vi "TestStand, Set Step Limits.vi"(6 "TS index":i32, 8 "error in":errorcluster, 10 "CDT_type":T1={"Measurement Name"="Signal_1", "Result"=3.0, "Low Limit"=-5.0, "High Limit"=5.0, "Units"="mV", "Comp"="GELE", "DataFmt"="%.3f", "LimitFmt"="%.4f"} {"Result" format="%.3g"; "High Limit" format="%.3g"; "Low Limit" format="%.3g"}, 11 "Sequence Context":refnum<k7>) -> (0 "error out":errorcluster, 3 "Sequence Context Out":refnum<k7>)   [LabVIEW 2010]
doc: "Sets TestStand Multiple Numeric Test properties for the following:\n\nRunState.Step.Result.Measurement[index]\nRunState.Step.Result.Measurement[index].Limits.High\nRunState.Step.Result.Measurement[index].Limits.Low\nRunState.Step.Result.Measurement[index].Limits.Units\nRunState.Step.Result.Measurement[index].Limits.Comp"
uses:
  TestStand_Result Control.ctl
  <vilib>/addons/TestStand/_TSUtility.llb/TestStand - Get Property Value (Object).vi
  <vilib>/addons/TestStand/_TSUtility.llb/TestStand - Set Property Value (String).vi
  <vilib>/addons/TestStand/_TSUtility.llb/TestStand - Set Property Value (Number).vi
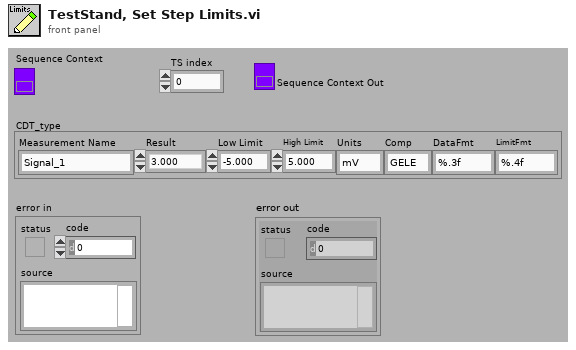
[diagram p1: front panel]
types:
  T1 = typedef "TestStand_Result Control.ctl" = cluster{"Measurement Name":string, "Result":dbl, "Low Limit":dbl, "High Limit":dbl, "Units":string, "Comp":string, "DataFmt":string, "LimitFmt":string}
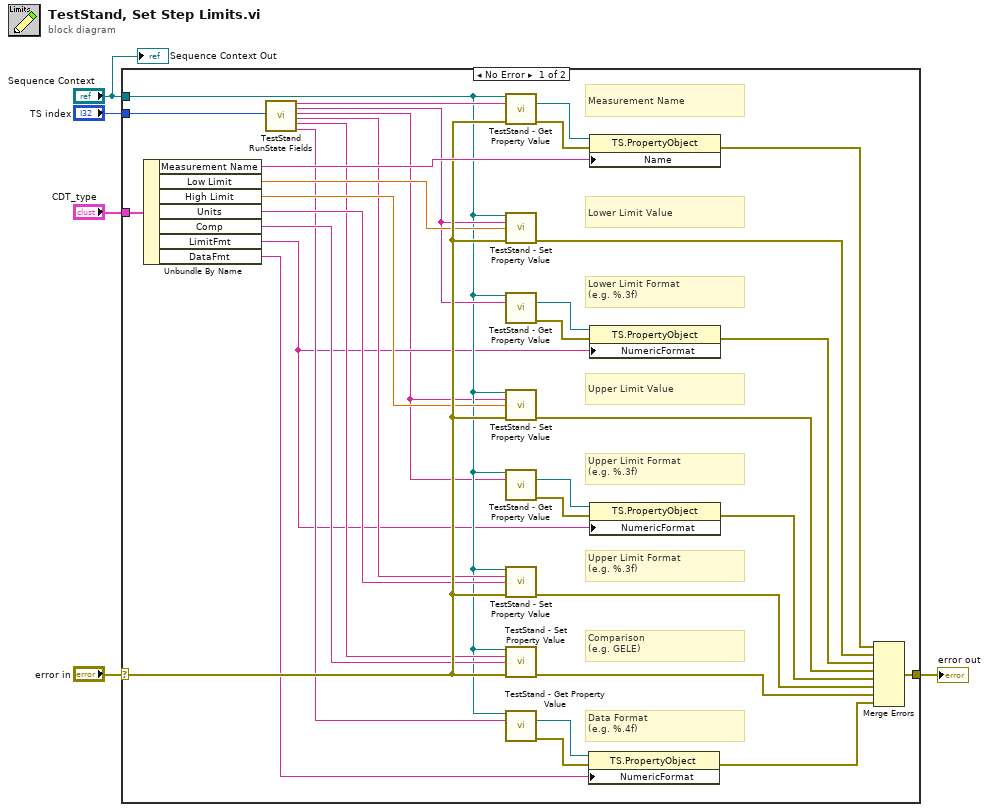
[diagram p0: block diagram]
diagram:
  n1 = case shown="No Error" "error in" {
    selector: "error in" -> [w32 w40]
    tunnel: [w34 w40] -> w5
    tunnel: "Sequence Context" -> [w12 _]
    tunnel: "CDT_type" -> [w33 _]
    tunnel: "TS index" -> [w23 _]
    frame No Error {
      # "Data Format\n(e.g. %.4f)"
      # "Comparison\n(e.g. GELE)"
      # "Upper Limit Format\n(e.g. %.3f)"
      # "Upper Limit Format\n(e.g. %.3f)"
      # "Upper Limit Value"
      # "Lower Limit Format\n(e.g. %.3f)"
      # "Lower Limit Value"
      # "Measurement Name"
      n2 = Unbundle By Name(w33) -> ("Measurement Name"=w39:string, "Low Limit"=w30:dbl, "High Limit"=w29:dbl, "Units"=w28:string, "Comp"=w27:string, "LimitFmt"=w11:string, "DataFmt"=w10:string)
      n3 = call "TestStand RunState Fields.vi"("index"=w23) -> ("Measurement Name"=w26:string, "Low Limit"=w19:string, "High Limit"=w9:string, "Units"=w25:string, "Comp"=w24:string, "Data"=w16:string)  [unwired: 13 in]
      n4 = call-poly <vilib>:"TestStand - Get Property Value.vi"("Sequence Context In"=w12, "Lookup String"=w26, "error in (no error)"=w32) -> ("Value"=w8:refnum<k7>, "error out"=w7:errorcluster)  [unwired: 10 in, 1 out]
      n5 = call-poly <vilib>:"TestStand - Set Property Value.vi"("Sequence Context In"=w12, "Lookup String"=w19, "New Value"=w30, "error in (no error)"=w32) -> ("error out"=w38:errorcluster)  [unwired: 10 in, 1 out]
      n6 = call-poly <vilib>:"TestStand - Get Property Value.vi"("Sequence Context In"=w12, "Lookup String"=w19) -> ("Value"=w22:refnum<k7>, "error out"=w20:errorcluster)  [unwired: 11 in, 1 out]
      n7 = call-poly <vilib>:"TestStand - Set Property Value.vi"("Sequence Context In"=w12, "Lookup String"=w9, "New Value"=w29, "error in (no error)"=w32) -> ("error out"=w35:errorcluster)  [unwired: 10 in, 1 out]
      n8 = call-poly <vilib>:"TestStand - Get Property Value.vi"("Sequence Context In"=w12, "Lookup String"=w9) -> ("Value"=w6:refnum<k7>, "error out"=w17:errorcluster)  [unwired: 11 in, 1 out]
      n9 = call-poly <vilib>:"TestStand - Set Property Value.vi"("Sequence Context In"=w12, "Lookup String"=w25, "New Value"=w28, "error in (no error)"=w32) -> ("error out"=w36:errorcluster)  [unwired: 10 in, 1 out]
      n10 = call-poly <vilib>:"TestStand - Set Property Value.vi"("Sequence Context In"=w12, "Lookup String"=w24, "New Value"=w27, "error in (no error)"=w32) -> ("error out"=w37:errorcluster)  [unwired: 10 in, 1 out]
      n11 = call-poly <vilib>:"TestStand - Get Property Value.vi"("Sequence Context In"=w12, "Lookup String"=w16) -> ("Value"=w21:refnum<k7>, "error out"=w13:errorcluster)  [unwired: 11 in, 1 out]
      n12 = property class="TS.PropertyObject"(reference=w21, error in=w13, "NumericFormat"=w10) -> (error out=w14:errorcluster)  [unwired: 1 out]
      n13 = property class="TS.PropertyObject"(reference=w8, error in=w7, "Name"=w39) -> (error out=w31:errorcluster)  [unwired: 1 out]
      n14 = property class="TS.PropertyObject"(reference=w22, error in=w20, "NumericFormat"=w11) -> (error out=w18:errorcluster)  [unwired: 1 out]
      n15 = property class="TS.PropertyObject"(reference=w6, error in=w17, "NumericFormat"=w11) -> (error out=w15:errorcluster)  [unwired: 1 out]
      n16 = Merge Errors(w31, w38, w18, w35, w15, w36, w37, w14) -> (w34:errorcluster)
    }
    frame Error {
    }
  }
  "error out" <- w5
  "Sequence Context Out" <- "Sequence Context"
